vi "启动参数选择.vi"() -> (2 "check？":bool, 3 "启动参数输出":T1)   [LabVIEW 2016]
uses:
  PLC/control/switch.ctl
  PLC/PLC.lvlib
panel:
  in  "取消":T2
  in  "确定":T2
  in  "启动参数":T1
  # "请选择需要启动的参数"
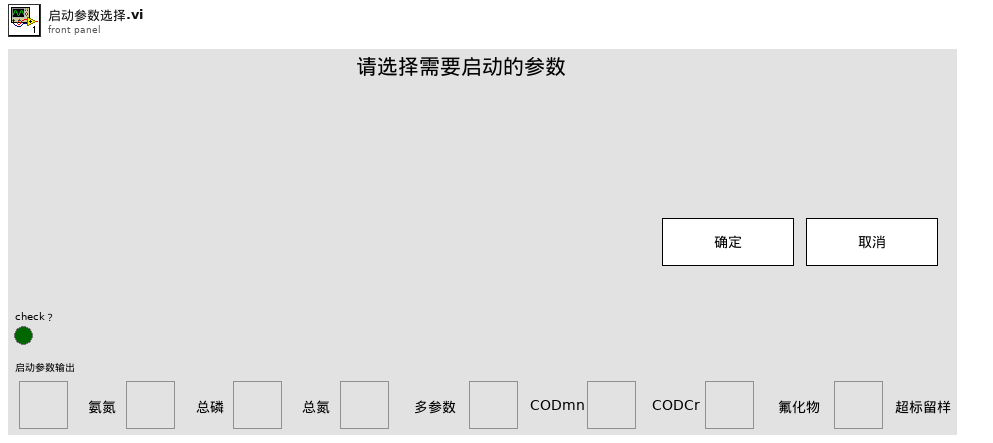
[diagram p1: front panel]
types:
  T1 = typedef "启动参数.ctl" = cluster{"氨氮":bool, "总磷":bool, "总氮":bool, "多参数":bool, "CODmn":bool, "CODCr":bool, "氟化物":bool, "超标留样启用":bool}
  T2 = typedef "PLC.lvlib/switch.ctl" = bool
  T3 = typedef "模块配置类型.ctl" = enum16{"单模块", "总磷总氮二合一模块", "氨氮总磷二合一模块"}
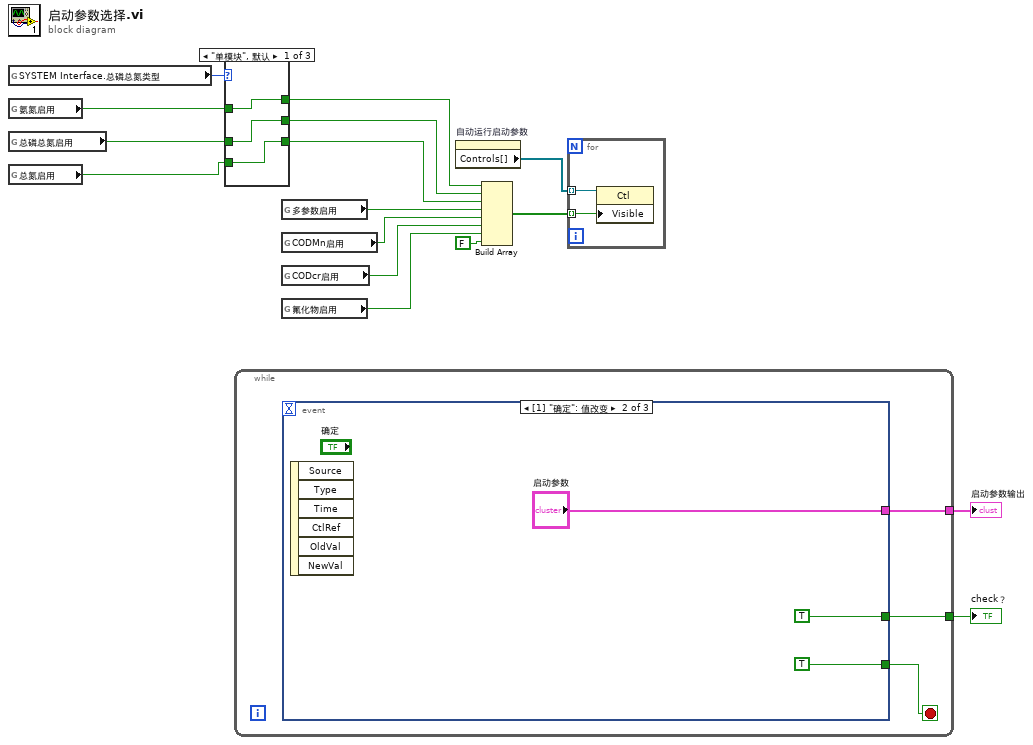
[diagram p0: block diagram]
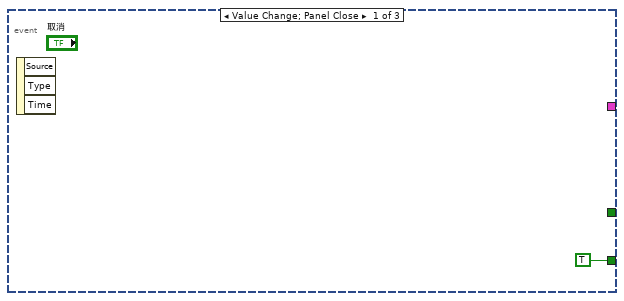
[diagram p2: hidden frame]
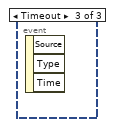
[diagram p3: hidden frame]
diagram:
  n1 = global read "系统设置全局变量.vi" "SYSTEM Interface.总磷总氮类型"() -> (w15:T3)
  n2 = global read "系统设置全局变量.vi" "氨氮启用"() -> (w14:bool)
  n3 = global read "系统设置全局变量.vi" "总磷总氮启用"() -> (w12:bool)
  n4 = global read "系统设置全局变量.vi" "总氮启用"() -> (w13:bool)
  n5 = case shown="\"单模块\", 默认" w15 {
    tunnel: [w17 w21 w23] -> w10
    tunnel: [w18 w21 w22] -> w9
    tunnel: [w19 w20 w23] -> w11
    tunnel: w14 -> [w19 w20 w23]
    tunnel: w13 -> [w18 _ w22]
    tunnel: w12 -> [w17 w21 _]
    frame "单模块", Default {
    }
    frame "总磷总氮二合一模块" {
    }
    frame "氨氮总磷二合一模块" {
    }
  }
  n6 = while {
    tunnel: [w26] -> w1
    tunnel: [w24] -> w2
    stop <- w25 stop-if-true
    n7 = event shown="[1] \"确定\": 值改变" {
      selector: _ -> [_ _ _]
      dyn-events: _ -> [_ _ _]
      timeout: _ -> [_ _ _]
      tunnel: [_ "启动参数" _] -> w26
      tunnel: [TRUE TRUE _] -> w25
      tunnel: [_ TRUE _] -> w24
      event Value Change; Panel Close {
        n8 = event-data() -> ()  [unwired: 1 in, 3 out]
      }
      event Value Change {
        n9 = event-data() -> ()  [unwired: 1 in, 6 out]
      }
      event Timeout {
        n10 = event-data() -> ()  [unwired: 1 in, 3 out]
      }
    }
  }
  "check？" <- w2
  "启动参数输出" <- w1
  n11 = global read "系统设置全局变量.vi" "多参数启用"() -> (w8:bool)
  n12 = global read "系统设置全局变量.vi" "CODMn启用"() -> (w7:bool)
  n13 = global read "系统设置全局变量.vi" "CODcr启用"() -> (w6:bool)
  n14 = global read "系统设置全局变量.vi" "氟化物启用"() -> (w5:bool)
  n15 = property on="自动运行启动参数" class="Clust (严格)"() -> ("Controls[]"=w16:refnum<vi>[])  [unwired: 2 in, 2 out]
  n16 = Build Array(w11, w10, w9, w8, w7, w6, w5, FALSE ("可见")) -> (w3:bool[])
  n17 = for {
    tunnel: w16 -> [w32] mode=indexing
    tunnel: w3 -> [w31] mode=indexing
    n18 = property class="Ctl"(reference=w32, "Visible"=w31) -> ()  [unwired: 1 in, 2 out]
  }
